vi "SubSystems.vi"(8 "error in":errorcluster) -> ()   [LabVIEW 2015]
doc: "This VI calls the various robot subsystems that will then run in parallel. New subSystems will automatlically script code to make the call."
uses:
  <vilib>/Rock Robotics/WPI/Camera/WPI_CameraImageSize.ctl
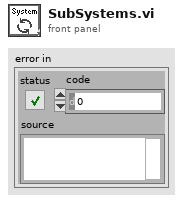
[diagram p1: front panel]
types:
  T1 = typedef "WPI_CameraImageSize.ctl" = enum16{"640x480", "320x240", "160x120", "Custom"}
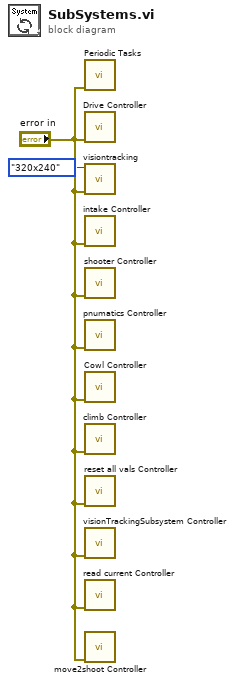
[diagram p0: block diagram]
diagram:
  n1 = call "Periodic Tasks.vi"("error in"="error in") -> ()  [unwired: 1 in, 10 out]
  n2 = call "Drive Controller.vi"("error in"="error in") -> ()  [unwired: 11 in]
  n3 = call "visiontracking.vi"("error in (no error)"="error in", "Image Size"=WPI_CameraImageSize."320x240") -> ()  [unwired: 6 in]
  n4 = call "intake Controller.vi"("error in"="error in") -> ()  [unwired: 11 in]
  n5 = call "shooter Controller.vi"("error in"="error in") -> ()  [unwired: 11 in]
  n6 = call "pnumatics Controller.vi"("error in"="error in") -> ()  [unwired: 11 in]
  n7 = call "Cowl Controller.vi"("error in"="error in") -> ()  [unwired: 11 in]
  n8 = call "climb Controller.vi"("error in"="error in") -> ()  [unwired: 11 in]
  n9 = call "reset all vals Controller.vi"("error in"="error in") -> ()  [unwired: 11 in]
  n10 = call "visionTrackingSubsystem Controller.vi"("error in"="error in") -> ()  [unwired: 11 in]
  n11 = call "read current Controller.vi"("error in"="error in") -> ()  [unwired: 11 in]
  n12 = call "move2shoot Controller.vi"("error in"="error in") -> ()  [unwired: 11 in]
